vi "Cast EtherCAT Data.vi"(11 "System State In":map{string, dbl}(c390)) -> (3 "System State Out":map{string, dbl}(c390))   [LabVIEW 2024, in "Hardware Controller.lvlib"]
uses:
  Hardware Controller.lvlib
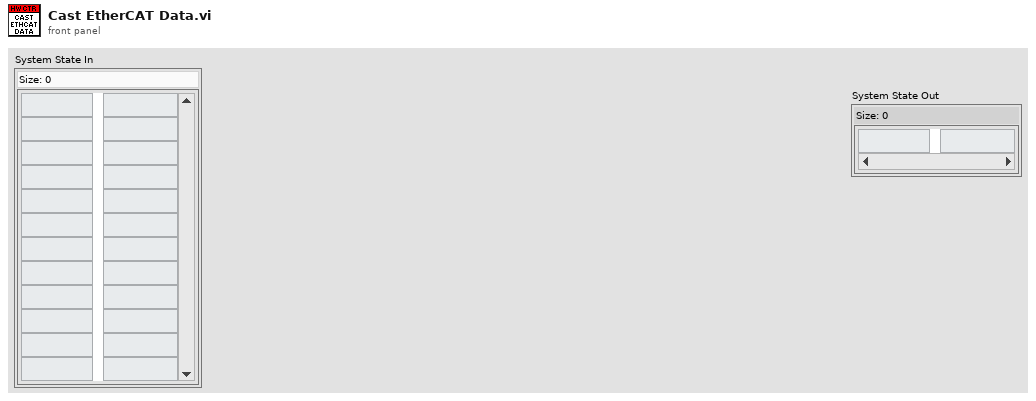
[diagram p1: front panel]
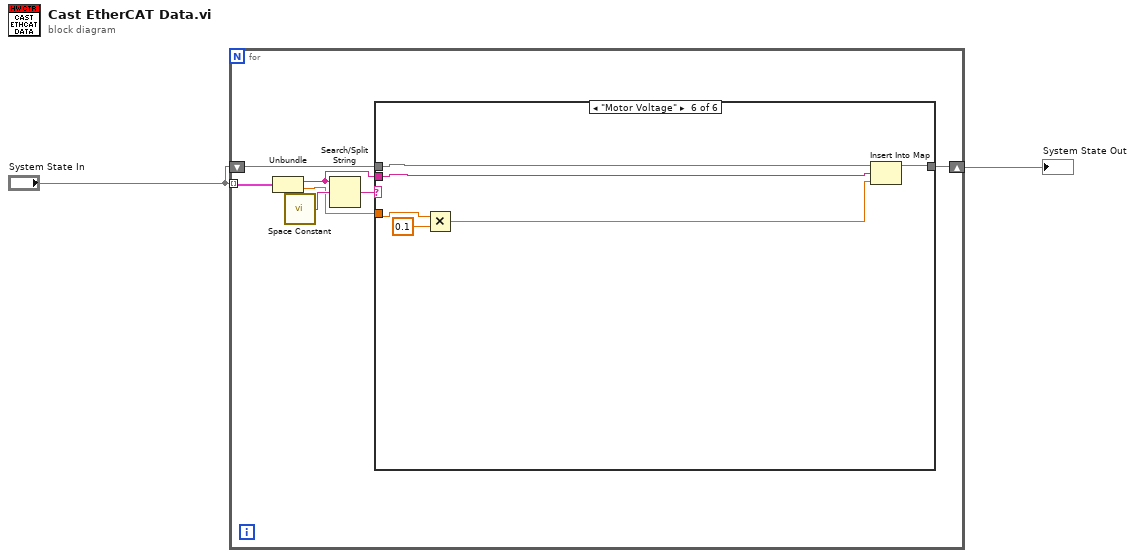
[diagram p0: block diagram]
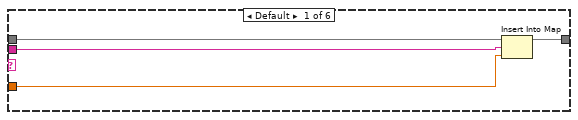
[diagram p2: hidden frame]
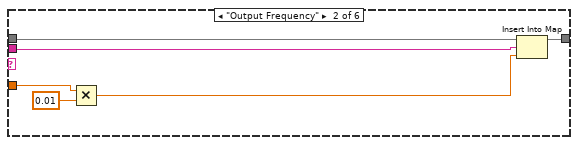
[diagram p3: hidden frame]
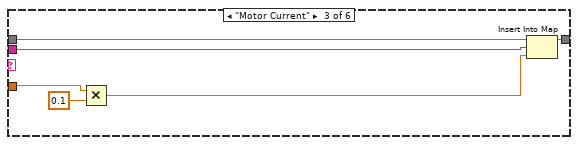
[diagram p4: hidden frame]
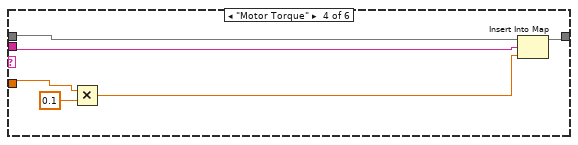
[diagram p5: hidden frame]
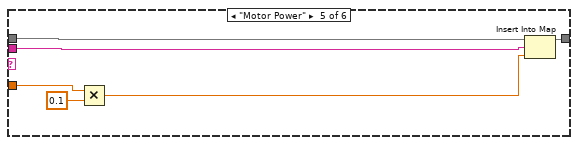
[diagram p6: hidden frame]
diagram:
  n1 = for {
    tunnel: "System State In" -> [w9] mode=indexing
    shift-right: [w3] -> w2
    shift-left: "System State In" -> [w6]
    n2 = Unbundle(w9) -> (w5:string, w4:dbl)
    n3 = call <vilib>:"Space Constant.vi"() -> ("String"=w8:string)
    n4 = Search/Split String(string=w5, search string/char (-)=w8) -> (match + rest of string=w7:string)  [unwired: 1 in, 2 out]
    n5 = case shown="\"Motor Voltage\"" w7 {
      tunnel: w6 -> [w12 w18 w21 w28 w35 w40]
      tunnel: w5 -> [w11 w17 w22 w27 w34 w39]
      tunnel: w4 -> [w10 w16 w23 w26 w33 w38]
      tunnel: [w13 w19 w20 w29 w32 w41] -> w3
      frame Default {
        n6 = Insert Into Map(map in=w12, key=w11, value=w10) -> (map out=w13:map{string, dbl})  [unwired: 2 out]
      }
      frame "Output Frequency" {
        n7 = Multiply(x=w16, y=0.01) -> (x*y=w14:dbl)
        n8 = Insert Into Map(map in=w18, key=w17, value=w14) -> (map out=w19:map{string, dbl})  [unwired: 2 out]
      }
      frame "Motor Current" {
        n9 = Multiply(x=w23, y=0.1) -> (x*y=w24:dbl)
        n10 = Insert Into Map(map in=w21, key=w22, value=w24) -> (map out=w20:map{string, dbl})  [unwired: 2 out]
      }
      frame "Motor Torque" {
        n11 = Multiply(x=w26, y=0.1) -> (x*y=w30:dbl)
        n12 = Insert Into Map(map in=w28, key=w27, value=w30) -> (map out=w29:map{string, dbl})  [unwired: 2 out]
      }
      frame "Motor Power" {
        n13 = Multiply(x=w33, y=0.1) -> (x*y=w36:dbl)
        n14 = Insert Into Map(map in=w35, key=w34, value=w36) -> (map out=w32:map{string, dbl})  [unwired: 2 out]
      }
      frame "Motor Voltage" {
        n15 = Multiply(x=w38, y=0.1) -> (x*y=w42:dbl)
        n16 = Insert Into Map(map in=w40, key=w39, value=w42) -> (map out=w41:map{string, dbl})  [unwired: 2 out]
      }
    }
  }
  "System State Out" <- w2
